vi "General PID Simulator.vi"() -> ()   [LabVIEW 2017]
doc: "This example demonstrates how to simulate a general PID controller."
uses:
  <vilib>/addons/control/pid/pid.llb/PID (DBL).vi
  <vilib>/addons/control/pid/NI_PID_pid.lvlib
  <vilib>/addons/control/pid/NI_PID_autopid.lvlib
panel:
  in  "autotune? (F)":bool
  out "tuning completed?":bool
  out "tuned PID gains":T1={"proportional gain (Kc)"=1.0, "integral time (Ti, min)"=0.01, "derivative time (Td, min)"=0.0} {"derivative time (Td, min)" format="%#.6g"; "integral time (Ti, min)" format="%#.6g"; "proportional gain (Kc)" format="%#.6g"}
  out "Manipulated variable":dbl(graph)
  in  "SP:":dbl(slide)=43.790849673202615 min=0.0 max=0.0 scale=0.0..100.0
  out "MV:":dbl(slide)=18.78965245852964 scale=-100.0..100.0
  out "PV:":dbl(slide)=60.754431603254424 scale=0.0..100.0
  in  "PID gains":T1={"proportional gain (Kc)"=20.0, "integral time (Ti, min)"=0.008, "derivative time (Td, min)"=0.001} {"derivative time (Td, min)" format="%.3f"; "integral time (Ti, min)" format="%.3f"; "proportional gain (Kc)" format="%.3f"}
  in  "Stop":bool
  out "Process variable and Setpoint":cluster{"initial PV":dbl, "SP:":dbl}(graph)
  # "Overview: This example demonstrates how to simulate a simple PID loop controller.\nInstructions:\n1. Run the VI and observe the Process variable (PV) following the Setpoint (SP) value while the output of the controller, also called Manipulated variable (MV), changes to keep both values near each other.\n2. After it settles down (value of PV and SP are near each other), change SP. You can just move the 'blue' arrow on the indicator. The MV will change to drive PV to SP again.\n3. Click Stop to stop the VI."
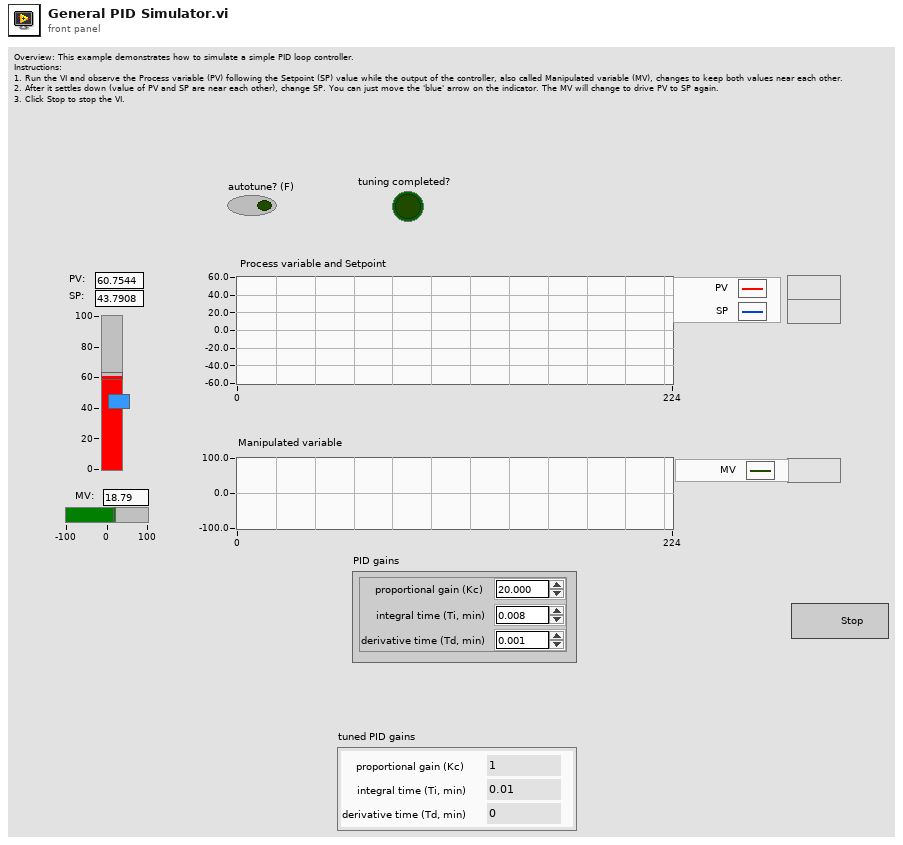
[diagram p1: front panel]
types:
  T1 = cluster{"proportional gain (Kc)":dbl, "integral time (Ti, min)":dbl, "derivative time (Td, min)":dbl}
  T2 = cluster{"static gain":dbl, "lag (min)":dbl, "dead cycles":dbl, "load %":dbl, "deadband":dbl, "noise level %":dbl, "initial PV":dbl, "initial PV 2":dbl}
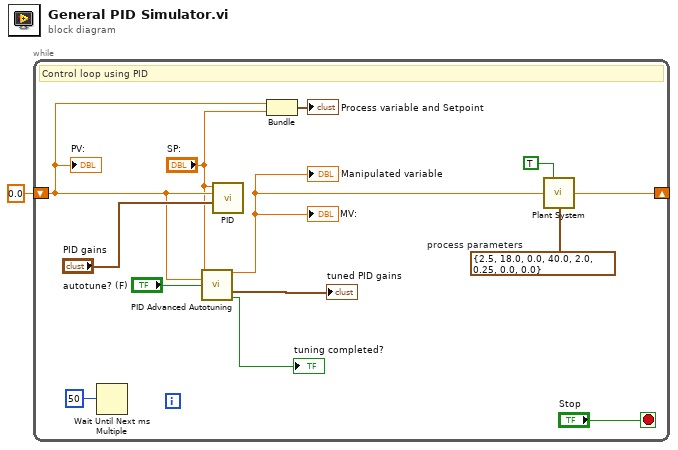
[diagram p0: block diagram]
diagram:
  n1 = while {
    shift-left: 0.0 ("Plant Output") -> [w7]
    shift-right: [w13] -> _
    stop <- "Stop" stop-if-true
    w9 = T2 {"static gain"=2.5, "lag (min)"=18.0, "dead cycles"=0.0, "load %"=40.0, "deadband"=2.0, "noise level %"=0.25, "initial PV"=0.0, "initial PV 2"=0.0}  # process parameters
    # "Control loop using PID"
    n2 = Wait Until Next ms Multiple(millisecond multiple=u32 50 ("unsigned 32bit integer")) -> ()  [unwired: 1 out]
    n3 = call <vilib>:"PID Advanced Autotuning.vi"("setpoint"="SP:", "process variable"=w7, "autotune? (F)"="autotune? (F)") -> ("output"=w5:dbl, "tuned PID gains"=→"tuned PID gains":T1, "tuning completed?"=→"tuning completed?":bool)  [unwired: 10 in]
    "MV:" <- w5
    "Manipulated variable" <- w5
    n4 = call-poly <vilib>:"PID.vi"("PID gains"="PID gains", "process variable"=w7, "setpoint"="SP:") -> ()  [unwired: 7 in, 2 out]
    n5 = Bundle("Plant Output"=w7, "SP:"="SP:") -> (→"Process variable and Setpoint":cluster{"Plant Output":dbl, "SP:":dbl})  [unwired: 1 in]
    n6 = call "Plant System.vi"("Integrator ?"=TRUE, "Plant Input"=w5, "process parameters"=w9) -> ("Plant Output"=w13:dbl)  [unwired: 12 in]
    "PV:" <- w7
  }
